vi "Submit Query.vi"() -> ()   [LabVIEW 2018]
uses:
  Collaborator/Command Configuration.ctl
  Collaborator/Collaborator.lvlib
panel:
  in  "error in (no error)":errorcluster
  out "Data out":string[](array[string])
  out "error out":errorcluster
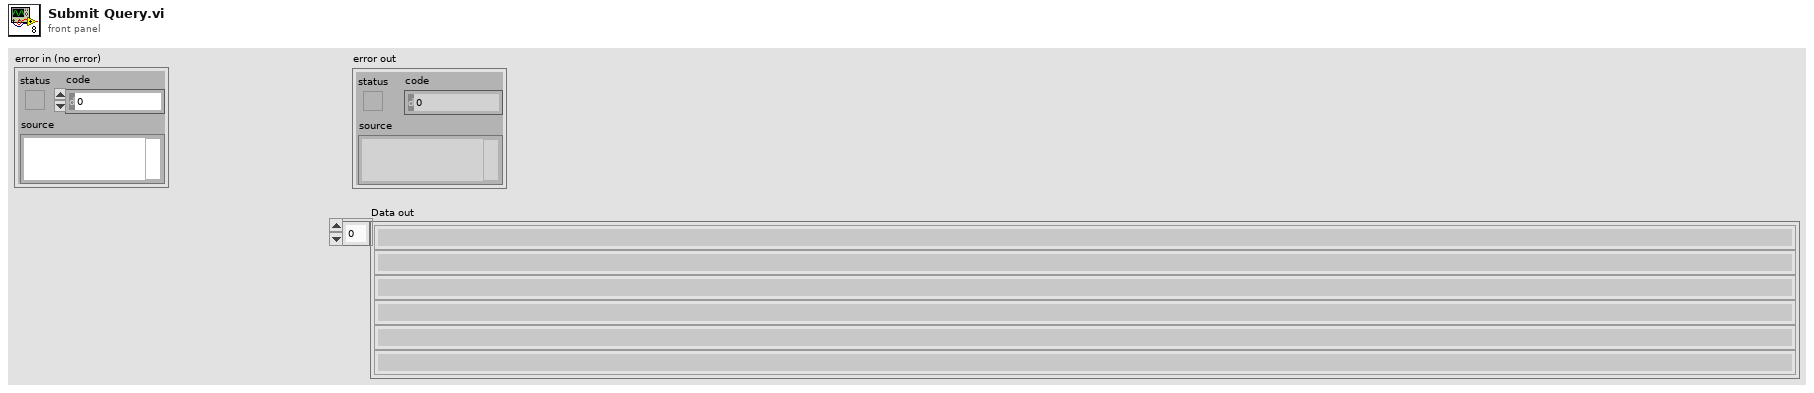
[diagram p1: front panel]
types:
  T1 = typedef "Command Configuration.ctl" = cluster{"Interface Name":string, "Method Name":string, "Arguments":cluster{"Argument Name":string, "Argument Value":string}[]}
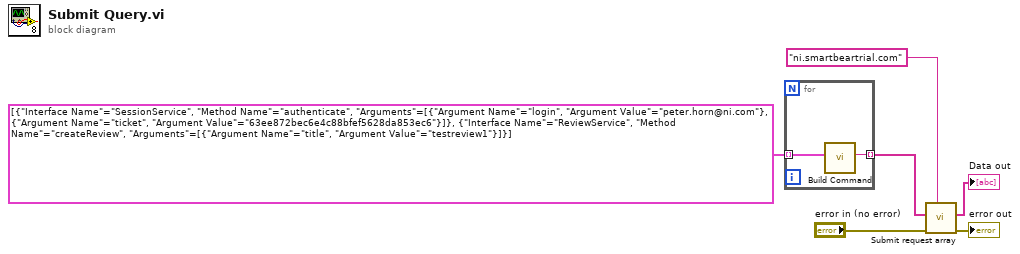
[diagram p0: block diagram]
diagram:
  n1 = for {
    tunnel: [w8] -> w2 mode=indexing
    tunnel: T1[] [{"Interface Name"="SessionService", "Method Name"="authenticate", "Arguments"=[{"Argument Name"="login", "Argument Value"="peter.horn@ni.com"}, {"Argument Name"="ticket", "Argument Value"="63ee872bec6e4c88bfef5628da853ec6"}]}, {"Interface Name"="ReviewService", "Method Name"="createReview", "Arguments"=[{"Argument Name"="title", "Argument Value"="testreview1"}]}] ("Array") -> [w7] mode=indexing
    n2 = call "Build Command.vi"("Command Definition"=w7) -> ("Command"=w8:string)  [unwired: 10 in]
  }
  n3 = call "Submit request array.vi"("Server Address"="ni.smartbeartrial.com", "error in (no error)"="error in (no error)", "Request Array"=w2) -> ("error out"=→"error out":errorcluster, "Return Data Array"=→"Data out":string[])  [unwired: 6 in, 1 out]
